vi "DetectPlatformType.vi"() -> (0 "Platform Type":T1)   [LabVIEW 2024, in "CustomActions.lvlib"]
uses:
  CustomActions.lvlib
  PlatformType--enum.ctl
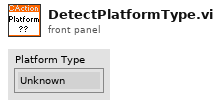
[diagram p1: front panel]
types:
  T1 = typedef "CustomActions.lvlib/PlatformType--enum.ctl" = enum16{"Unknown", "Win32", "Win64", "Linux64"}
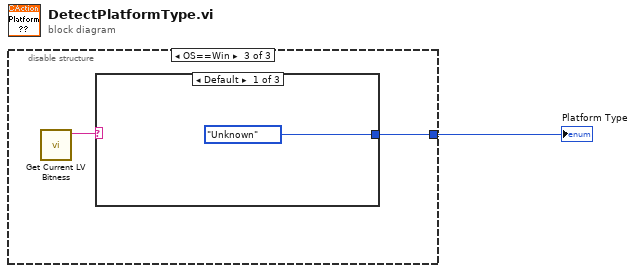
[diagram p0: block diagram]
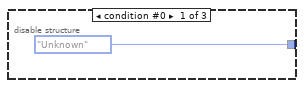
[diagram p2: hidden frame]
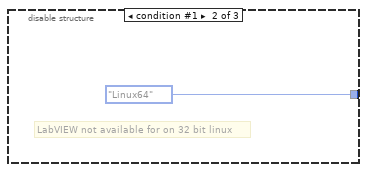
[diagram p3: hidden frame]
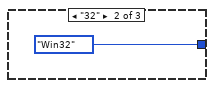
[diagram p4: hidden frame]
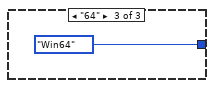
[diagram p5: hidden frame]
diagram:
  n1 = disable-structure shown="OS==Win" {
    disable-tunnel: [PlatformType--enum."Unknown" ("Platform Type") PlatformType--enum."Linux64" ("Platform Type") w4] -> w1
    frame condition #0 {
    }
    frame condition #1 {
      # "LabVIEW not available for on 32 bit linux"
    }
    frame condition #2 (active) {
      n2 = call <vilib>:"Get Current LV Bitness.vi"() -> ("bitness"=w5:string)  [unwired: 11 in]
      n3 = case shown="Default" w5 {
        tunnel: [PlatformType--enum."Unknown" ("Platform Type") PlatformType--enum."Win32" ("Platform Type") PlatformType--enum."Win64" ("Platform Type")] -> w4
        frame Default {
        }
        frame "32" {
        }
        frame "64" {
        }
      }
    }
  }
  "Platform Type" <- w1
